vi "CH_LM Measurement Initiate.vi"(0 "Meter Index":i32, 5 "error in (no error)":errorcluster, 7 "Timeout / ms (3000)":i32=3000, 9 "Lock Timeout / ms (1000)":i32=1000) -> (11 "Lock timed out":bool, 14 "Meter Index":i32, 19 "error out":errorcluster)   [LabVIEW 2017, in "CH_LM.lvlib"]
doc: "This VI enables the streaming mode.\n\nThe streaming data is send with approximatly 10 Hz from LabMax and must be read with CH_LM Streaming Read Data.vi.\n\nStreaming Mode: Default: All Data; as set in the _CH_LM Default Instrument Setup.vi.\n\n<B>Hint:</B> The USB Binary Data Streaming will be enabled with this command."
uses:
  CH_LM.lvlib
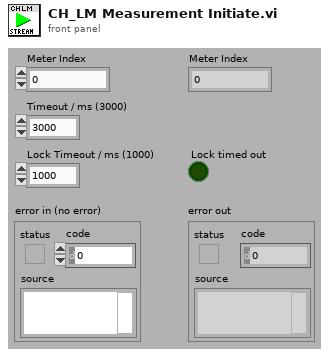
[diagram p1: front panel]
types:
  T1 = typedef "CH_LM.lvlib/CH_LM Communication Mode.ctl" = enum16{"None", "USB", "GPIB", "RS232"}
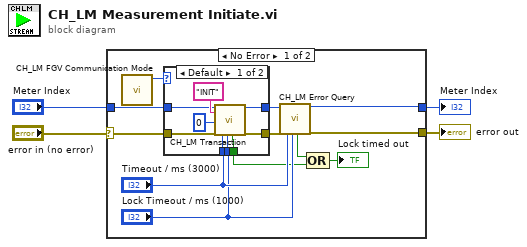
[diagram p0: block diagram]
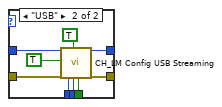
[diagram p2: hidden frame]
diagram:
  n1 = case shown="No Error" "error in (no error)" {
    selector: "error in (no error)" -> [w5 w36]
    tunnel: [w15 w36] -> w4
    tunnel: "Meter Index" -> [w6 w35]
    tunnel: [w16 w35] -> w1
    frame No Error {
      n2 = call "CH_LM FGV Communication Mode.vi"() -> ("Communication Mode"=w10:T1)  [unwired: 3 in, 5 out]
      n3 = case shown="Default" w10 {
        tunnel: w6 -> [w22 w34]
        tunnel: [w21 w29] -> w8
        tunnel: w5 -> [w19 w33]
        tunnel: [w20 w28] -> w7
        tunnel: "Timeout / ms (3000)" -> [w18 w32]
        tunnel: "Lock Timeout / ms (1000)" -> [w17 w27]
        tunnel: [w23 w26] -> w9
        frame Default {
          n4 = call "CH_LM Transaction.vi"("Meter Index"=w22, "Command String"="INIT", "NofStrings (-1:all)"=0, "error in (no error)"=w19, "Timeout / ms (3000)"=w18, "Lock Timeout / ms (1000)"=w17) -> ("Lock timed out"=w23:bool, "Meter Index"=w21:i32, "error out"=w20:errorcluster)  [unwired: 11 out]
        }
        frame "USB" {
          n5 = call "CH_LM Config USB Streaming.vi"("Meter Index"=w34, "USB Streaming (disable)"=TRUE, "error in (no error)"=w33, "Timeout / ms (3000)"=w32, "Action (query)"=TRUE, "Lock Timeout / ms (1000)"=w27) -> ("Lock timed out"=w26:bool, "Meter Index"=w29:i32, "error out"=w28:errorcluster)  [unwired: 11 out]
        }
      }
      n6 = call "CH_LM Error Query.vi"("Meter Index"=w8, "error in (no error)"=w7, "Timeout / ms (3000)"="Timeout / ms (3000)", "Lock Timeout / ms (1000)"="Lock Timeout / ms (1000)") -> ("Lock timed out"=w14:bool, "Meter Index"=w16:i32, "error out"=w15:errorcluster)  [unwired: 13 out]
      n7 = Compound Arithmetic op=OR(w14, w9) -> (→"Lock timed out":bool)
    }
    frame Error {
    }
  }
  "error out" <- w4
  "Meter Index" <- w1
